vi "GetSource.vi"(6 "error in":errorcluster, 9 "LeftShiftRegister in":refnum<class "LeftShiftRegister.lvclass">) -> (0 "error out":errorcluster, 3 "LeftShiftRegister out":refnum<class "LeftShiftRegister.lvclass">, 4 "name":string)   [LabVIEW 2014, in "Raspberry Pi Compatible Compiler for LabVIEW.lvlib" / "LeftShiftRegister.lvclass"]
uses:
  LeftShiftRegister.lvclass
  Tunnel/Tunnel.lvclass
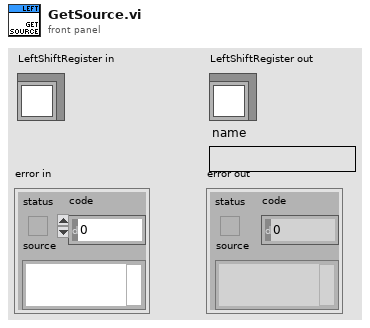
[diagram p1: front panel]
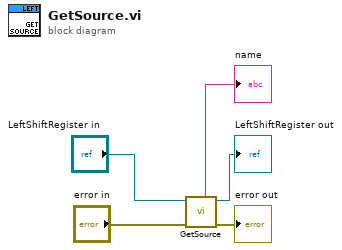
[diagram p0: block diagram]
diagram:
  n1 = call-parent "GetSource.vi"("error in"="error in", "Tunnel in"="LeftShiftRegister in") -> ("error out"=→"error out":errorcluster, "Tunnel out"=→"LeftShiftRegister out":refnum<class "LeftShiftRegister.lvclass">, "name"=→"name":string)  [unwired: 5 in]
